vi "Save_Channel_Config.vi"(8 "Error in":errorcluster, 10 "configuration file path":path, 11 "Channel_Information_Control":T1 {"Input Terminal Configuration" items=["default"=-1, "RSE"=10083, "NRSE"=10078, "Differential"=10106, "Pseudodifferential"=12529]}) -> (0 "error out":errorcluster)   [LabVIEW 2021]
doc: "Save the Channel Information to an XML Config File."
uses:
  typedef/Channel_Information_Control_array.ctl
  typedef/Channel_Information_Control_single.ctl
  <vilib>/Utility/config.llb/Write Key (String).vi
  <vilib>/Utility/config.llb/NI_LVConfig.lvlib
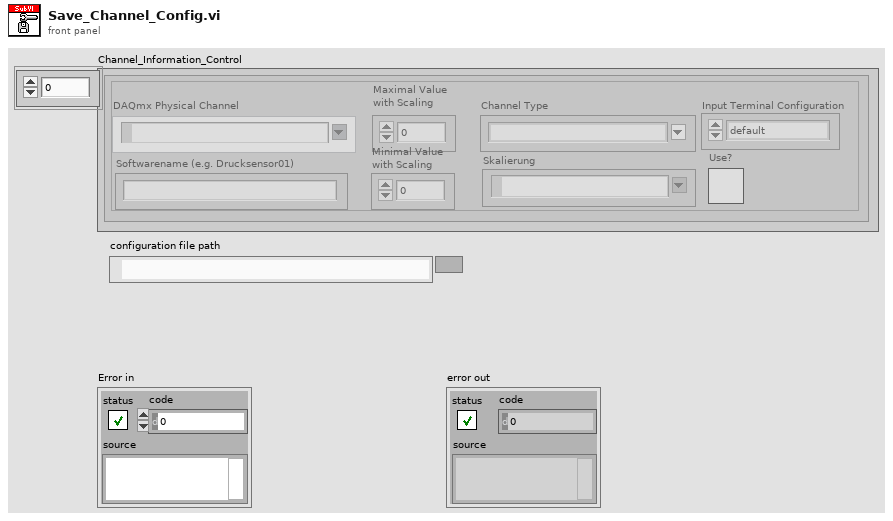
[diagram p1: front panel]
types:
  T1 = typedef "Channel_Information_Control_array.ctl" = T2[]
  T2 = typedef "Channel_Information_Control_single.ctl" = cluster{"DAQmx Physical Channel":tag, "Softwarename (e.g. Drucksensor01)":string, "Maximal Value \nwith Scaling":dbl, "Minimal Value\nwith Scaling":dbl, "Channel Type":string, "Input Terminal Configuration":i32, "Skalierung":tag, "Use?":bool}
  T3 = typedef "NI_LVConfig.lvlib/Config Data RefNum.ctl" = refnum<k1>
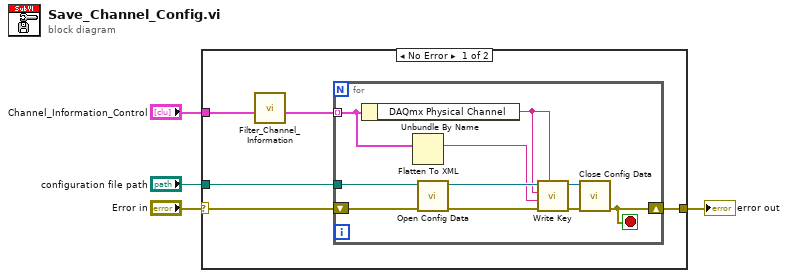
[diagram p0: block diagram]
diagram:
  n1 = case shown="No Error" "Error in" {
    selector: "Error in" -> [w7 w20]
    tunnel: "configuration file path" -> [w9 _]
    tunnel: "Channel_Information_Control" -> [w6 _]
    tunnel: [w8 w20] -> w3
    frame No Error {
      n2 = call "Filter_Channel_Information.vi"("Channel_Information_Control"=w6) -> ("Array"=w5:T2[])  [unwired: 10 in]
      n3 = for {
        tunnel: w9 -> [w12]
        tunnel: w5 -> [w11] mode=indexing
        shift-right: [w10] -> w8
        shift-left: w7 -> [w13]
        stop <- w10 stop-if-true
        n4 = Unbundle By Name(w11) -> ("DAQmx Physical Channel"=w16:tag)
        n5 = Flatten To XML(6:w11) -> (2:w18:string)
        n6 = call <vilib>:"Open Config Data.vi"("error in (no error)"=w13, "configuration file path"=w12) -> ("error out"=w17:errorcluster, "refnum"=w19:T3)  [unwired: 7 in, 1 out]
        n7 = call-poly <vilib>:"Write Key.vi"("section"=w16, "error in (no error)"=w17, "value"=w18, "key"=w16, "refnum"=w19) -> ("error out"=w14:errorcluster, "refnum out"=w15:T3)  [unwired: 4 in, 1 out]
        n8 = call <vilib>:"Close Config Data.vi"("error in (no error)"=w14, "refnum"=w15) -> ("error out"=w10:errorcluster)  [unwired: 8 in, 1 out]
      }
    }
    frame Error {
    }
  }
  "error out" <- w3
